vi "save as csv.vi"(8 "error in (no error)":errorcluster, 10 "Data":string[][](array[string]), 11 "generic data log in":refnum<class "generic data log.lvclass">) -> (0 "error out":errorcluster, 3 "generic data log out":refnum<class "generic data log.lvclass">)   [LabVIEW 2025, in "Data Log.lvlib" / "generic data log.lvclass"]
uses:
  generic data log.lvclass
  generic data log.lvclass/generic data log.ctl
  <vilib>/Utility/file.llb/Write Delimited Spreadsheet (string).vi
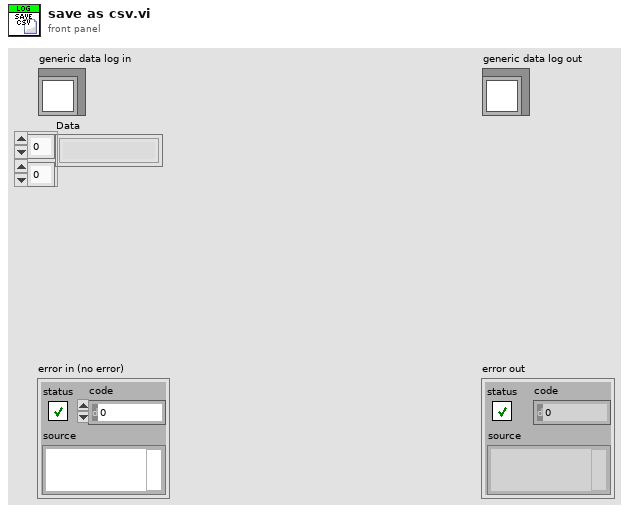
[diagram p1: front panel]
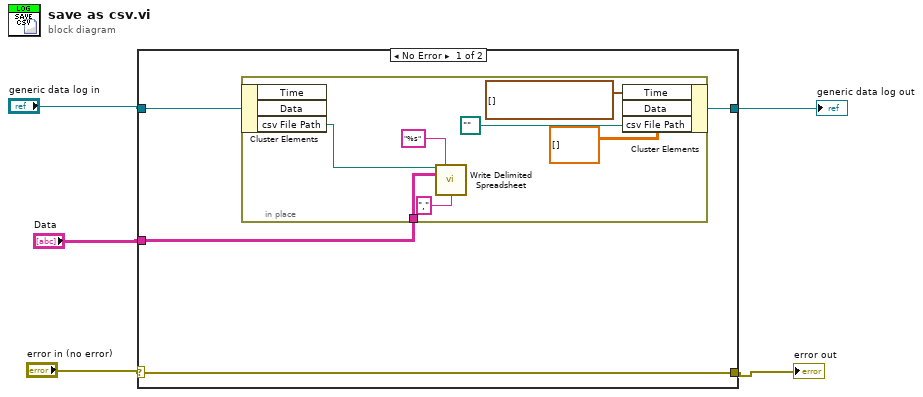
[diagram p0: block diagram]
diagram:
  n1 = case shown="No Error" "error in (no error)" {
    selector: "error in (no error)" -> [w9 w18]
    tunnel: [w9 w18] -> w2
    tunnel: [w7 w17] -> w4
    tunnel: "generic data log in" -> [w8 w17]
    tunnel: "Data" -> [w6 _]
    frame No Error {
      n2 = in-place {
        in-place-border: w6 -> [w13]
        n3 = in-place-cluster #1(w8) -> ("csv File Path"=w11:path)  [unwired: 2 out]
        n4 = call-poly <vilib>:"Write Delimited Spreadsheet.vi"("file path (dialog if empty)"=w11, "format (%s)"="%s", "2D data"=w13, "delimiter (\\t)"="," ("delimiter (\\t)")) -> ()  [unwired: 10 in, 2 out]
        n5 = in-place-cluster #1("Time"=timestamp[] [] ("Data.Time"), "Data"=dbl[][] [] ("Data.Data"), "csv File Path"=path "") -> (w7:refnum<class "generic data log.lvclass">)
      }
    }
    frame Error {
    }
  }
  "error out" <- w2
  "generic data log out" <- w4
